vi "Graph - XY Map-01237.vi"() -> ()   [LabVIEW 2011]
doc: "Sample numeric display item."
uses:
  <vilib>/NI Veristand/Display Template Support/Display Template Support.llb/cluster_Screen Item Settings.ctl
  <vilib>/NI Veristand/Display Template Support/Display Template Support.llb/cluster_Graph Scale Settings.ctl
  <vilib>/NI Veristand/Display Template Support/Display Template Support.llb/cluster_Graph Plot Settings.ctl
  <vilib>/NI Veristand/Display Template Support/Display Template Support.llb/cluster_Graph Handler Message.ctl
  <vilib>/NI Veristand/Display Template Support/Display Template Support.llb/enum_Graph Handler Message.ctl
  <vilib>/NI Veristand/Display Template Support/Display Template Support.llb/sub_Display Template Handler Graph.vi
  <vilib>/NI Veristand/Display Template Support/Display Template Support.llb/sub_Display Template Data Handler Graph.vi
panel:
  out "XY Graph":cluster{dbl[], dbl[]}(graph)
  out "Graph":waveform(dbl)[](graph)
  out "Label":string="Numeric"
  in  "Once":bool
  out "Y.Autoscale":bool
  in  "Y.Scale.Auto":bool
  out "X.Autoscale":bool
  in  "X.Scale.Auto":bool
  in  "Legend":bool
  in  "Setup":bool
  in  "Hold":bool
  in  "Item.Data":T1
  # "Autoscale"
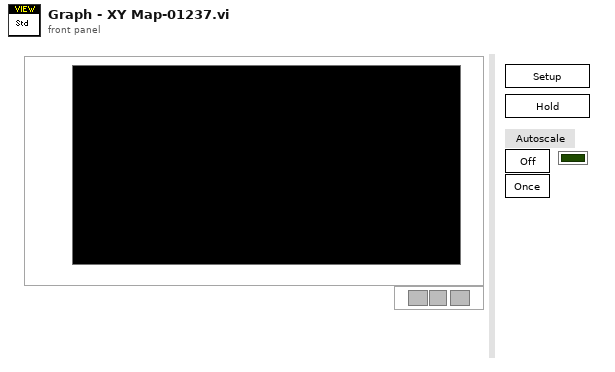
[diagram p1: front panel]
types:
  T1 = typedef "cluster_Screen Item Settings.ctl" = cluster{"Template VI":string, "Position X":i32, "Position Y":i32, "Custom":string, "Show Title Bar":bool, "ID":i32, "Always On Top":bool, "Allow Resize":bool, "Allow Minimize":bool, "Allow Close":bool, "Size to Screen":bool, "Screen.ID":i32, "State":enum16{"Normal", "New"}, "Title":string, "Window Bounds":cluster{"[0]":i16, "[1]":i16, "[2]":i16, "[3]":i16}, "Channel Ref":u64, "Unit":string, "Default Units?":bool, "Flash Limit?":bool, "Color 1":u32, "Color 2":u32, "Color 3":u32, "Color 4":u32, "Bck Color":u32, "Fore Color":u32, "Limit 1":dbl, "Limit 2":dbl, "Limit 3":dbl, "Limit 4":dbl, "Limit Mode 1":i32, "Limit Mode 2":i32, "Limit Mode 3":i32, "Limit Mode 4":i32, "Scale Precision":i32, "Scale Min":dbl, "Scale Max":dbl, "Format":i32, "Precision":i32, "Background Type":i32, "IDs":i32[], "Units":string[], "Labels":string[], "Scale Factor":dbl, "Scale Offset":dbl, "YScale Index":u32[], "XScale":T2, "YScales":T2[], "Plots":T3[], "Update Period":dbl, "History Length":dbl, "My.Ref":refnum<vi>, "Is Control?":bool, "Channel Paths":string[], "Custom Data":variant}
  T2 = typedef "cluster_Graph Scale Settings.ctl" = cluster{"Format":u8, "Precision":u8, "Fit":u8, "Label":string, "Use Default Label":bool, "Label Visible":bool, "Min":dbl, "Max":dbl}
  T3 = typedef "cluster_Graph Plot Settings.ctl" = cluster{"Bar Style":u8, "Fill To":i16, "Fill/PtColor":u32, "Line Style":u8, "Line Width":u8, "Color":u32, "Interp":u8, "Point Style":u8}
  T4 = cluster{"xmin":dbl, "xmax":dbl, "ymin":dbl, "ymax":dbl, "xinc":dbl, "yinc":dbl, "pixellg2":dbl}
  T5 = typedef "cluster_Graph Handler Message.ctl" = cluster{"Message":T6, "Data":variant}
  T6 = typedef "enum_Graph Handler Message.ctl" = enum16{"None", "Stop", "Hold", "Update Channels", "New Settings", "Control Value", "Edit Value"}
  T7 = typedef "LVBoundsTypeDef.ctl" = cluster{"Width":u32, "Height":u32}
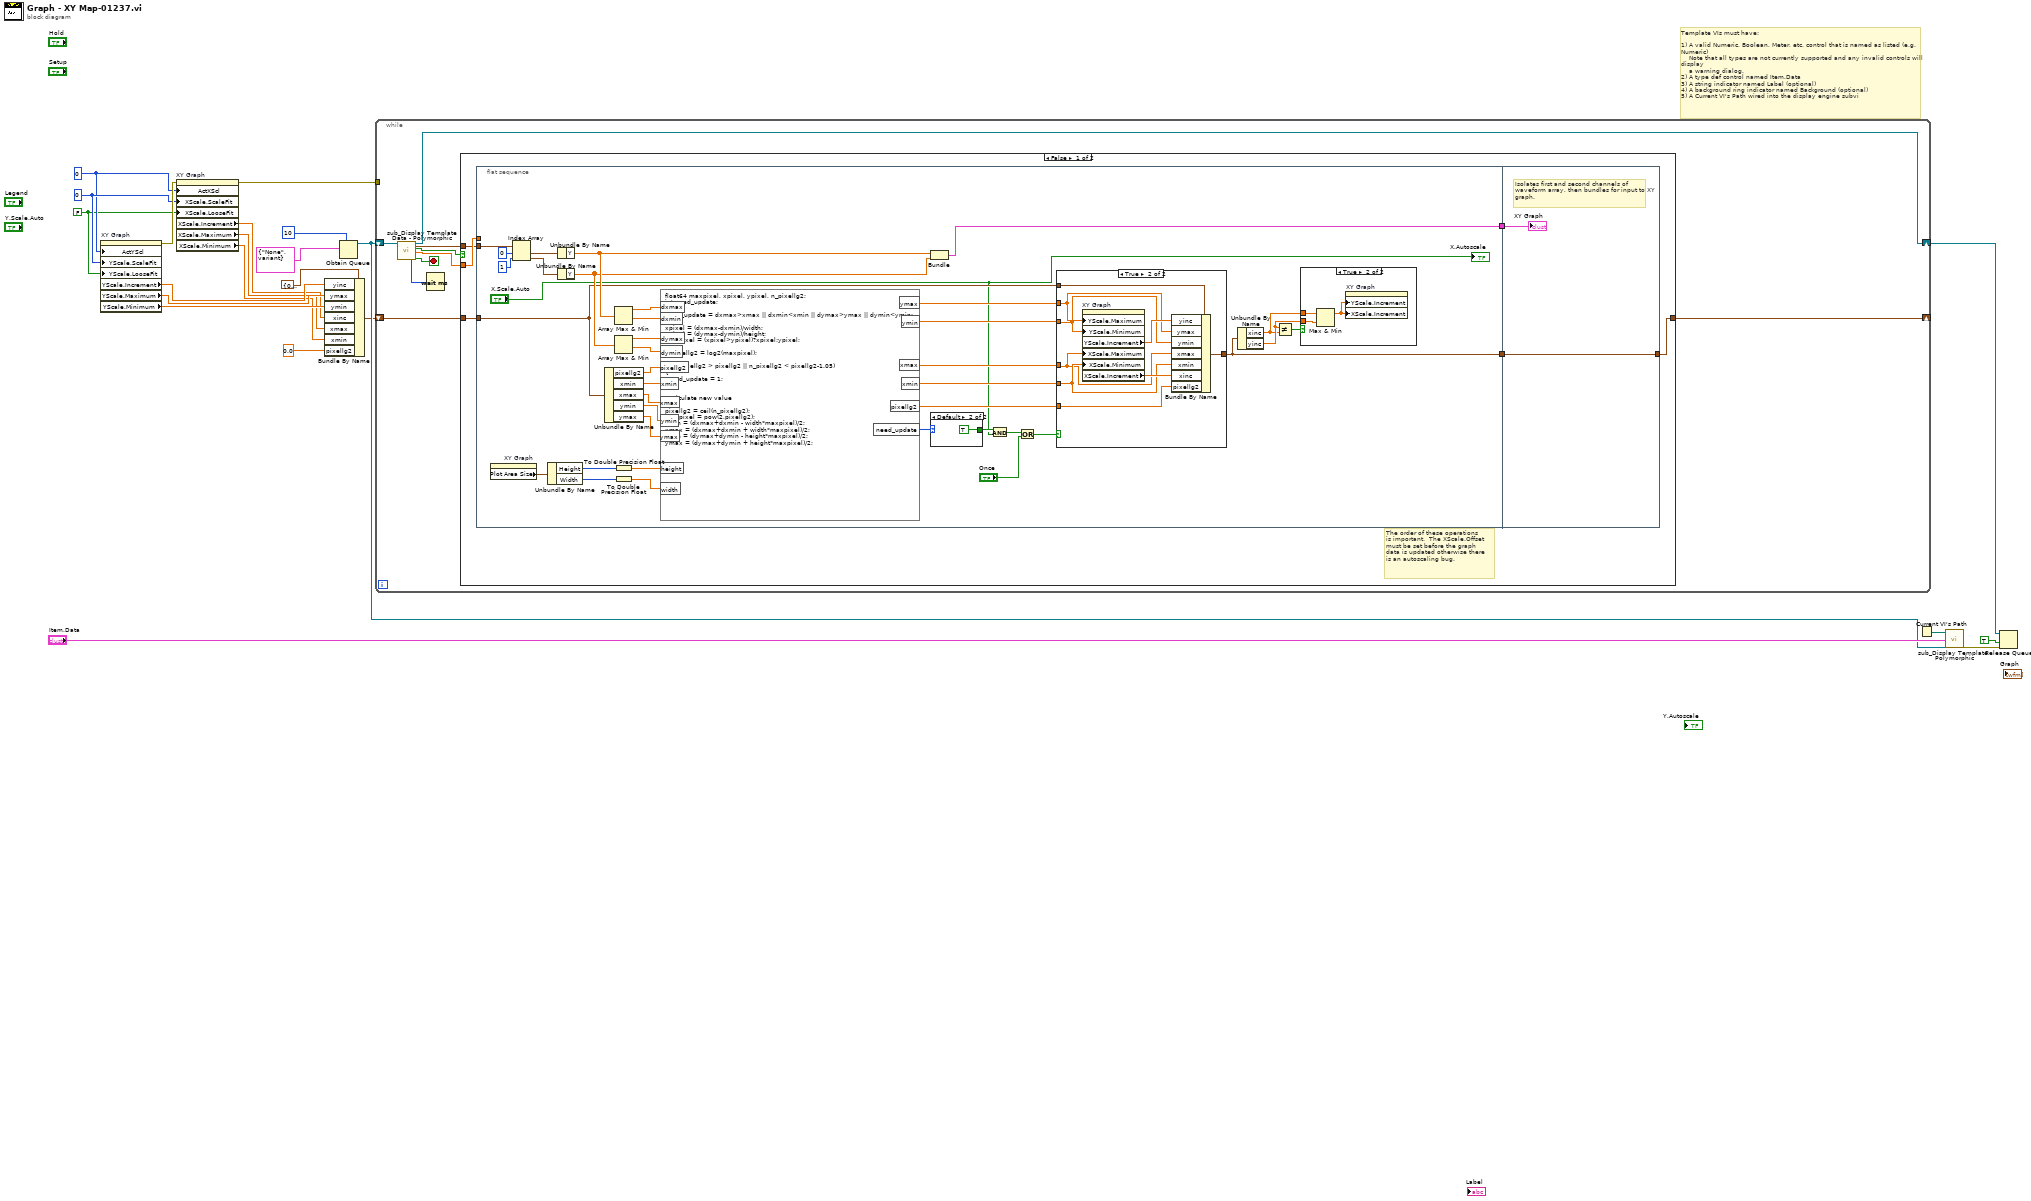
[diagram p0: block diagram]
diagram:
  w10 = FALSE
  w13 = u8 0 ("Y Scale.Scale Fit")
  w12 = 0 ("Active Y Scale")
  # "Template VIs must have:\n\n1) A valid Numeric, Boolean, Meter, etc. control that is named as listed (e.g. Numeric)\n    Note that all types are not currently supported and any invalid controls will display\n    a warning dialog.\n2) A type def control named Item.Data\n3) A string indicator named Label (optional)\n4) A background ring indicator named Background (optional)\n5) A Current VI's Path wired into the display engine subvi"
  n1 = property on="XY Graph" class="XYGraph (strict)"("ActYScl"=w12, "YScale.ScaleFit"=w13, "YScale.LooseFit"=w10) -> (error out=w14:errorcluster, "YScale.Increment"=w8:dbl, "YScale.Maximum"=w7:dbl, "YScale.Minimum"=w6:dbl)  [unwired: 2 in, 1 out]
  n2 = property on="XY Graph" class="XYGraph (strict)"(error in=w14, "ActXScl"=w12, "XScale.ScaleFit"=w13, "XScale.LooseFit"=w10) -> (error out=w11:errorcluster, "XScale.Increment"=w5:dbl, "XScale.Maximum"=w4:dbl, "XScale.Minimum"=w3:dbl)  [unwired: 1 in, 1 out]
  n3 = Bundle By Name(cluster=T4 {"xmin"=0.0, "xmax"=0.0, "ymin"=0.0, "ymax"=0.0, "xinc"=0.0, "yinc"=0.0, "pixellg2"=0.0} ("Cluster"), "yinc"=w8, "ymax"=w7, "ymin"=w6, "xinc"=w5, "xmax"=w4, "xmin"=w3, "pixellg2"=0.0) -> (w9:T4)
  n4 = Obtain Queue(max queue size (-1, unlimited)=10, element data type=T5 {"Message"=enum."None", "Data"=variant} ("Message")) -> (queue out=w16:refnum<queue>)  [unwired: 2 in, 3 out]
  n5 = while {
    shift-right: [w31] -> w20
    shift-left: w16 -> [w30]
    tunnel: w11 -> [_]
    shift-right: [w23] -> _
    shift-left: w9 -> [w24]
    stop <- w25 stop-if-true
    n6 = call-poly <vilib>:"sub_Display Template Data - Polymorphic.vi"("queue"=w30) -> ("Wait.Time"=w28:u32, "queue out"=w31:refnum<queue>, "Graph.Data"=w29:waveform(dbl)[], "Hold"=w26:bool, "XScale.Offset"=w27:dbl, "Stop"=w25:bool)  [unwired: 13 out]
    n7 = Wait (ms)(milliseconds to wait=w28) -> ()  [unwired: 1 out]
    n8 = case shown="False" w26 {
      tunnel: w27 -> [w37 _]
      tunnel: w29 -> [w36 _]
      tunnel: w24 -> [w34 w92]
      tunnel: [w32 w92] -> w23
      frame False {
        # "The order of these operations\nis important.  The XScale.Offset\nmust be set before the graph\ndata is updated otherwise there\nis an autoscaling bug."
        n9 = flat-sequence {
          tunnel: w37 -> [_]
          tunnel: w36 -> [w67]
          tunnel: [w68] -> w35
          tunnel: w34 -> [w60]
          tunnel: [w40] -> w33
          tunnel: w35 -> [w91]
          tunnel: w33 -> [w90]
          tunnel: [w90] -> w32
          frame #0 {
            n10 = property on="XY Graph" class="XYGraph (strict)"() -> ("Plot Area Size"=w75:T7)  [unwired: 2 in, 2 out]
            n11 = Index Array(array=w67, index #1=0 ("index"), index #2=1 ("index")) -> (element #1=w71:waveform(dbl), element #2=w72:waveform(dbl))
            n12 = Unbundle By Name(w75) -> ("Height"=w74:u32, "Width"=w73:u32)
            n13 = Unbundle By Name(w71) -> ("Y"=w66:dbl[])
            n14 = Unbundle By Name(w72) -> ("Y"=w65:dbl[])
            n15 = Unbundle By Name(w60) -> ("pixellg2"=w48:dbl, "xmin"=w51:dbl, "xmax"=w52:dbl, "ymin"=w49:dbl, "ymax"=w50:dbl)
            n16 = Array Max & Min(array=w66) -> (max value=w54:dbl, min value=w53:dbl)  [unwired: 2 out]
            n17 = Array Max & Min(array=w65) -> (max value=w56:dbl, min value=w55:dbl)  [unwired: 2 out]
            n18 = To Double Precision Float(number=w74) -> (double precision float=w47:dbl)
            n19 = To Double Precision Float(number=w73) -> (double precision float=w46:dbl)
            n20 = formula code="float64 maxpixel, xpixel, ypixel, n_pixellg2;\nint need_update;\n\nneed_update = dxmax>xmax || dxmin<xmin || dymax>ymax || dymin<ymin;\n\nxpixel = (dxmax-dxmin)/width;\nypixel = (dymax-dymin)/height;\nmaxpixel = (xpixel>ypixel)?xpixel:ypixel;\n\nn_pixellg2 = log2(maxpixel);\n\nif( n_pixellg2 > pixellg2 || n_pixellg2 < pixellg2-1.05)\n{\n\tneed_update = 1;\n}\n\n//calculate new value\n\npixellg2 = ceil(n_pixellg2);\nmaxpixel = pow(2,pixellg2);\nxmin = (dxmax+dxmin - width*maxpixel)/2;\nxmax = (dxmax+dxmin + width*maxpixel)/2;\nymin = (dymax+dymin - height*maxpixel)/2;\nymax = (dymax+dymin + height*maxpixel)/2;"("dxmax"=w54, "dxmin"=w53, "dymax"=w56, "dymin"=w55, "xmax"=w52, "xmin"=w51, "ymax"=w50, "ymin"=w49, "pixellg2"=w48, "height"=w47, "width"=w46) -> ("xmax"=w43:dbl, "xmin"=w42:dbl, "ymax"=w59:dbl, "ymin"=w58:dbl, "pixellg2"=w57:dbl, "need_update"=w45:i32)
            n21 = Bundle("Y"=w66, "Y"=w65) -> (w68:cluster{"Y":dbl[], "Y":dbl[]})  [unwired: 1 in]
            n22 = case shown="Default" w45 {
              tunnel: [_ TRUE] -> w44
              frame 0 {
              }
              frame Default {
              }
            }
            n23 = Compound Arithmetic op=AND(w44, "X.Scale.Auto") -> (w61:bool)
            n24 = Or(x=w61, y="Once") -> (x .or. y?=w39:bool)
            n25 = case shown="True" w39 {
              tunnel: w58 -> [_ w85]
              tunnel: w59 -> [_ w86]
              tunnel: w60 -> [w80 w89]
              tunnel: [w80 w87] -> w40
              tunnel: w57 -> [_ w81]
              tunnel: w43 -> [_ w82]
              tunnel: w42 -> [_ w83]
              frame False {
              }
              frame True {
                n26 = property on="XY Graph" class="XYGraph (strict)"("YScale.Maximum"=w86, "YScale.Minimum"=w85, "XScale.Maximum"=w82, "XScale.Minimum"=w83) -> ("YScale.Increment"=w88:dbl, "XScale.Increment"=w84:dbl)  [unwired: 2 in, 2 out]
                n27 = Bundle By Name(cluster=w89, "yinc"=w88, "ymax"=w86, "ymin"=w85, "xmax"=w82, "xmin"=w83, "xinc"=w84, "pixellg2"=w81) -> (w87:T4)
              }
            }
            n28 = Unbundle By Name(w40) -> ("xinc"=w62:dbl, "yinc"=w63:dbl)
            n29 = Not Equal?(x=w63, y=w62) -> (x != y?=w64:bool)
            n30 = case shown="True" w64 {
              tunnel: w62 -> [_ w78]
              tunnel: w63 -> [_ w77]
              frame False {
              }
              frame True {
                n31 = Max & Min(x=w78, y=w77) -> (max(x,y)=w79:dbl)  [unwired: 1 out]
                n32 = property on="XY Graph" class="XYGraph (strict)"("YScale.Increment"=w79, "XScale.Increment"=w79) -> ()  [unwired: 2 in, 2 out]
              }
            }
            "X.Autoscale" <- "X.Scale.Auto"
          }
          frame #1 {
            # "Isolates first and second channels of waveform array, then bundles for input to XY graph."
            "XY Graph" <- w91
          }
        }
      }
      frame True {
      }
    }
  }
  n33 = Current VI's Path() -> (path=w22:path)
  n34 = call-poly <vilib>:"sub_Display Template - Polymorphic.vi"("Parent.Path"=w22, "Item.Data"="Item.Data", "queue"=w16) -> ("error out"=w15:errorcluster)  [unwired: 16 out]
  n35 = Release Queue(queue=w20, force destroy? (F)=TRUE, error in (no error)=w15) -> ()  [unwired: 3 out]
